vi "test_CCDDiscover.vi"() -> ()   [LabVIEW 2023]
uses:
  Classes/CCD/CCD.lvclass
  <vilib>/addons/_JKI Toolkits/Caraya/classes/Assert/Assert Not Error.vi
  <vilib>/addons/_JKI Toolkits/Caraya/classes/Assert/Assert Equal Value and Type_Variant.vi
  <vilib>/addons/_JKI Toolkits/Caraya/classes/Test/Test.lvclass
  <vilib>/addons/_JKI Toolkits/Caraya/classes/Assert/Assert.lvclass
  Libraries/DeviceManager/DeviceManager.lvlib
panel:
  out "error out":errorcluster
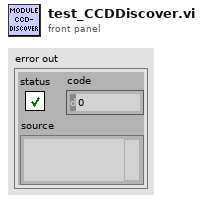
[diagram p1: front panel]
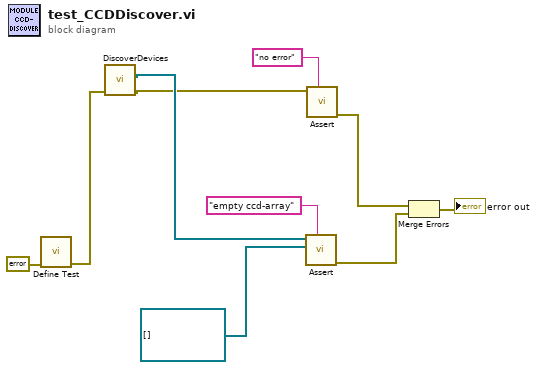
[diagram p0: block diagram]
diagram:
  n1 = call <vilib>:"Define Test.vi"("error in (no error)"=errorcluster {"status"=FALSE, "code"=0, "source"=""}) -> ("error out"=w8:errorcluster)  [unwired: 9 in, 1 out]
  n2 = call "DiscoverDevices.vi"("error in"=w8) -> ("error out"=w3:errorcluster, "CCDs"=w7:refnum<class "CCD.lvclass">[])  [unwired: 6 in, 3 out]
  n3 = call-poly <vilib>:"Assert.vi"("Label"="empty ccd-array" ("Label (VI Title)"), "Y"=refnum<class "CCD.lvclass">[] [] ("CCDs"), "X"=w7) -> ("error out"=w1:errorcluster)  [unwired: 7 in, 1 out]
  n4 = call-poly <vilib>:"Assert.vi"("Label"="no error" ("Label (VI Title)"), "Not Error?"=w3) -> ("error out"=w5:errorcluster)  [unwired: 8 in, 1 out]
  n5 = Merge Errors(w5, w1) -> (→"error out":errorcluster)
